vi "Convert Lidar Data to Cartesian.vi"(11 "Polar Lidar Data":cluster{dbl[], dbl[]}) -> (3 "Cartesian Lidar Data":cluster{"X":dbl, "Y":dbl}[](array[cluster]))   [LabVIEW 2017]
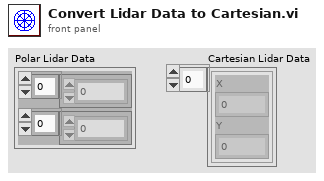
[diagram p1: front panel]
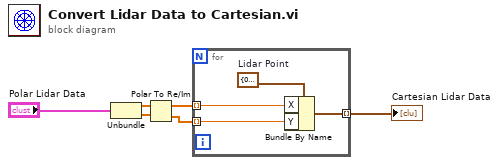
[diagram p0: block diagram]
diagram:
  n1 = Unbundle("Polar Lidar Data") -> (w2:dbl[], w3:dbl[])
  n2 = Polar To Re/Im(2:w3, 3:w2) -> (0:w5:dbl[], 1:w4:dbl[])
  n3 = for {
    tunnel: w4 -> [w9] mode=indexing
    tunnel: w5 -> [w8] mode=indexing
    tunnel: [w7] -> w6 mode=indexing
    w10 = cluster{"X":dbl, "Y":dbl} {"X"=0.0, "Y"=0.0}  # Lidar Point
    n4 = Bundle By Name(cluster=w10, "X"=w9, "Y"=w8) -> (w7:cluster{"X":dbl, "Y":dbl})
  }
  "Cartesian Lidar Data" <- w6
